vi "VL53L0X_SetLimitCheckRangeIgnoreThreshold.vi"(9 "Enable (T)":bool=TRUE, 10 "LimitCheckValue":u32, 11 "REV2mDistanceSensorDevRef":T1) -> (3 "REV2mDistanceSensorDevRef Out":T1)   [LabVIEW 2019, in "DistanceSensorDriver.lvlib"]
uses:
  DistanceSensorDriver.lvlib
  Typedef/REV2mDistanceSensorDevRef.ctl
  Typedef/Ports.ctl
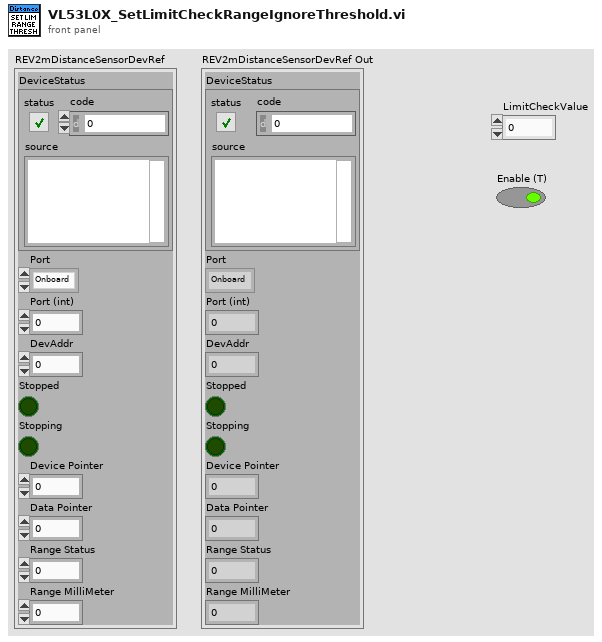
[diagram p1: front panel]
types:
  T1 = typedef "DistanceSensorDriver.lvlib/REV2mDistanceSensorDevRef.ctl" = cluster{"DeviceStatus":errorcluster, "Port":T2, "Port (int)":i32, "DevAddr":i32, "Stopped":bool, "Stopping":bool, "Device Pointer":u64, "Data Pointer":u64, "Range Status":u8, "Range MilliMeter":u16}
  T2 = typedef "DistanceSensorDriver.lvlib/Ports.ctl" = enum32{"Onboard", "MXP"}
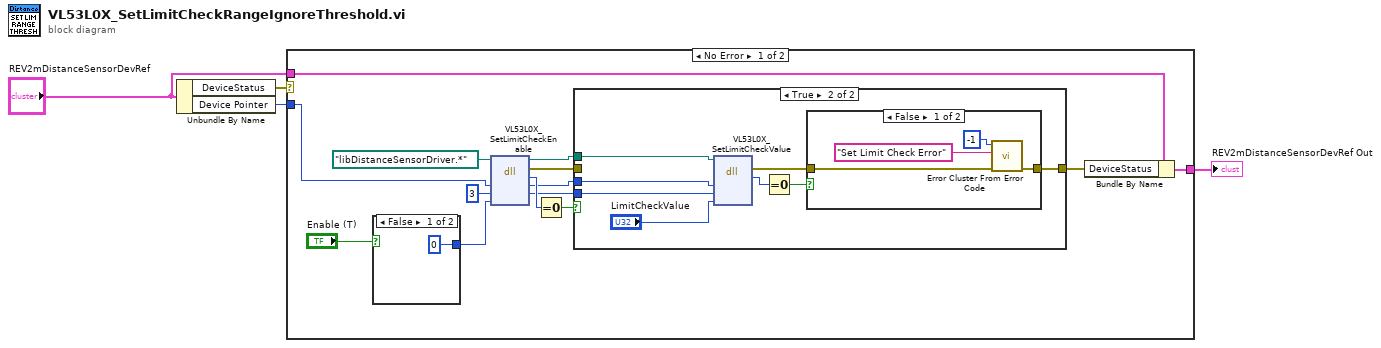
[diagram p0: block diagram]
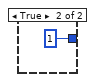
[diagram p2: hidden frame]
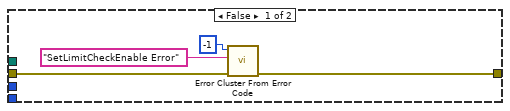
[diagram p3: hidden frame]
diagram:
  n1 = Unbundle By Name("REV2mDistanceSensorDevRef") -> ("DeviceStatus"=w1:errorcluster, "Device Pointer"=w4:u64)
  n2 = case shown="No Error" w1 {
    tunnel: w4 -> [w13 _]
    tunnel: [w12 w38] -> w3
    tunnel: "REV2mDistanceSensorDevRef" -> [w11 w38]
    frame No Error {
      n3 = case shown="False" "Enable (T)" {
        tunnel: [0 ("LimitCheckEnable") 1 ("LimitCheckEnable")] -> w5
        frame False {
        }
        frame True {
        }
      }
      n4 = dll-call lib="?" fn="VL53L0X_SetLimitCheckEnable"(path in=path "libDistanceSensorDriver.*", "Dev"=w13, "LimitCheckId"=u16 3, "LimitCheckEnable"=w5) -> (path out=w7:path, error out=w14:errorcluster, "Status"=w15:i32, "Dev"=w10:u64, "LimitCheckId"=w8:u16)  [unwired: 3 in]
      n5 = Equal To 0?(x=w15) -> (x = 0?=w18:bool)
      n6 = case shown="True" w18 {
        tunnel: w14 -> [w21 _]
        tunnel: [w24 w25] -> w17
        tunnel: w10 -> [_ w32]
        tunnel: w8 -> [_ w31]
        tunnel: w7 -> [_ w29]
        frame False {
          n7 = call <vilib>:"Error Cluster From Error Code.vi"("error in (no error)"=w21, "error message (\"\")"="SetLimitCheckEnable Error" ("error message (\"\")"), "error code (0)"=-1) -> ("error out"=w24:errorcluster)  [unwired: 6 in]
        }
        frame True {
          n8 = dll-call lib="?" fn="VL53L0X_SetLimitCheckValue"(path in=w29, "Dev"=w32, "LimitCheckId"=w31, "LimitCheckValue"="LimitCheckValue") -> (error out=w26:errorcluster, "Status"=w28:i32)  [unwired: 5 in, 1 out]
          n9 = Equal To 0?(x=w28) -> (x = 0?=w27:bool)
          n10 = case shown="False" w27 {
            tunnel: w26 -> [w34 w37]
            tunnel: [w33 w37] -> w25
            frame False {
              n11 = call <vilib>:"Error Cluster From Error Code.vi"("error in (no error)"=w34, "error message (\"\")"="Set Limit Check Error" ("error message (\"\")"), "error code (0)"=-1) -> ("error out"=w33:errorcluster)  [unwired: 6 in]
            }
            frame True {
            }
          }
        }
      }
      n12 = Bundle By Name(cluster=w11, "DeviceStatus"=w17) -> (w12:T1)
    }
    frame Error {
    }
  }
  "REV2mDistanceSensorDevRef Out" <- w3
